vi "Draw.vi"(8 "error in (no error)":errorcluster, 9 "DrawPoint(Ingored If Not Wired)":T1={"X"=-1, "Y"=-1}, 10 "PictureIn":picture, 11 "reference in":refnum<class "Row.lvclass">) -> (0 "error out":errorcluster, 1 "Width":i32, 2 "PictureOut":picture, 3 "reference in":refnum<class "Row.lvclass">)   [LabVIEW 2012, in "Row.lvclass"]
uses:
  Row.lvclass
  Glyph_class/Position.ctl
  Character_class/Character.lvclass
  Glyph_class/Glyph.lvclass
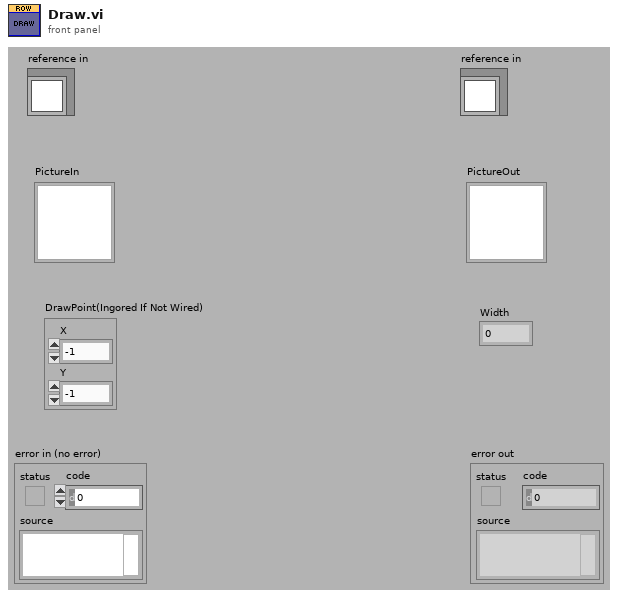
[diagram p1: front panel]
types:
  T1 = typedef "Glyph.lvclass/Position.ctl" = cluster{"X":i32, "Y":i32}
  T2 = typedef "Row.lvclass/ObjectAttributes.ctl" = cluster{"Characters":refnum<class "Character.lvclass">[], "StartPoint":T1, "CharacterSpacing":i32}
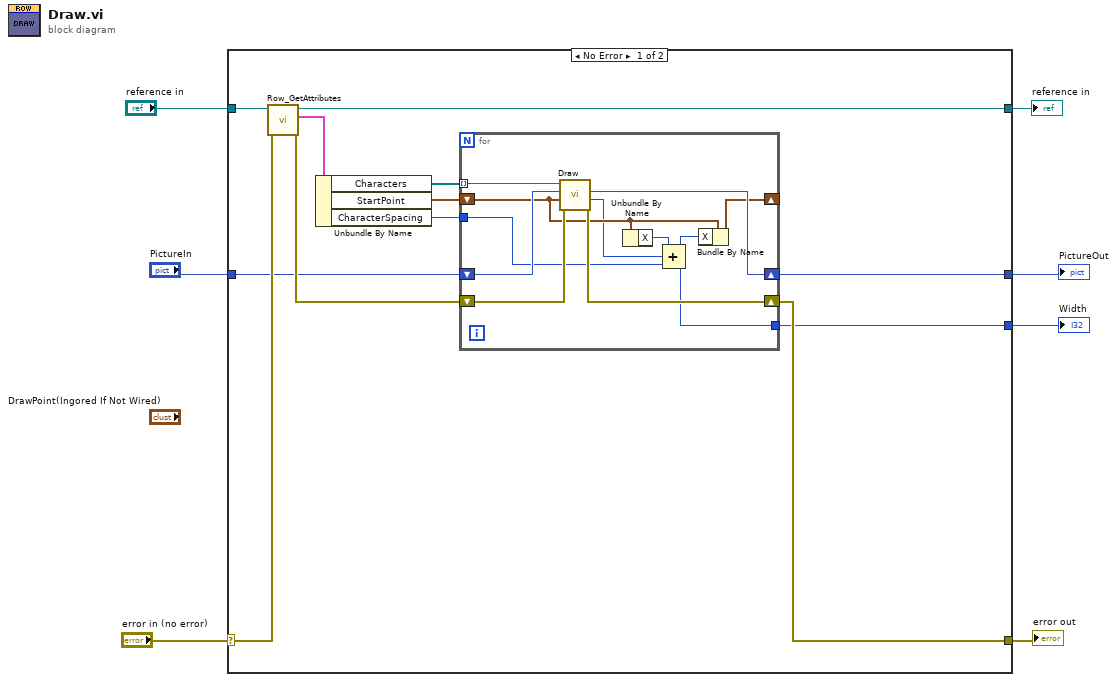
[diagram p0: block diagram]
diagram:
  n1 = case shown="No Error" "error in (no error)" {
    selector: "error in (no error)" -> [w19 w33]
    tunnel: [w13 w33] -> w6
    tunnel: [w16 w32] -> w4
    tunnel: "reference in" -> [w17 w32]
    tunnel: "PictureIn" -> [w12 w31]
    tunnel: [w11 w31] -> w2
    tunnel: [w8 _] -> w1
    frame No Error {
      n2 = call "Row_GetAttributes.vi"("error in (no error)"=w19, "reference in"=w17) -> ("error out"=w14:errorcluster, "Data"=w18:T2, "reference out"=w16:refnum<class "Row.lvclass">)  [unwired: 6 in, 1 out]
      n3 = Unbundle By Name(w18) -> ("Characters"=w15:refnum<class "Character.lvclass">[], "StartPoint"=w10:T1, "CharacterSpacing"=w9:i32)
      n4 = for {
        tunnel: w15 -> [w30] mode=indexing
        shift-right: [w28] -> w13
        shift-left: w14 -> [w29]
        shift-right: [w26] -> w11
        shift-left: w12 -> [w27]
        shift-right: [w21] -> _
        shift-left: w10 -> [w25]
        tunnel: w9 -> [w22]
        tunnel: [w20] -> w8
        n5 = call-dynamic "Draw.vi"("error in (no error)"=w29, "DrawPoint(Ingored If Not Wired)"=w25, "PictureIn"=w27, "reference in"=w30) -> ("error out"=w28:errorcluster, "Width"=w23:i32, "PictureOut"=w26:picture)  [unwired: 4 in, 1 out]
        n6 = Unbundle By Name(w25) -> ("X"=w24:i32)
        n7 = Compound Arithmetic op=ADD(w24, w23, w22) -> (w20:i32)
        n8 = Bundle By Name(cluster=w25, "X"=w20) -> (w21:T1)
      }
    }
    frame Error {
    }
  }
  "error out" <- w6
  "reference in" <- w4
  "PictureOut" <- w2
  "Width" <- w1
